vi "lab1AirheaterParams.vi"() -> ()   [LabVIEW 2019]
uses:
  Control 1.ctl
  <vilib>/Simulation/Scripting/Companion Diagram/SimConfigNode/SimParams.ctl
  <vilib>/Simulation/Scripting/Companion Diagram/SimConfigNode/_simSolvers.ctl
  <vilib>/Simulation/Implementation/Shared/SIMSCR Execution Mode.ctl
  <vilib>/Simulation/Param Hierarchy/Typedefs/SIMPH Param Control Actions.ctl
  <vilib>/Simulation/Implementation/Shared/NILVSim_ParamChanged.vi
  <vilib>/Simulation/Implementation/Shared/NILVSIM_BeginStep.vi
  <vilib>/Simulation/Implementation/Shared/NILVSim_Manager.vi
  <vilib>/Utility/error.llb/Clear Errors.vi
  <vilib>/Simulation/Implementation/Shared/NILVSim_FinalizeModel.vi
  <vilib>/DAQmx/write.llb/DAQmx Write (Analog DBL 1Chan 1Samp).vi
  <vilib>/DAQmx/read.llb/DAQmx Read (Analog DBL 1Chan 1Samp).vi
  <vilib>/Simulation/Implementation/Shared/SIM Unbundle Sim Info.vi
  <vilib>/Simulation/Implementation/Shared/NILVSim_Initialize.vi
  <vilib>/Simulation/Utility/Implementation/NILVSim Get Time and IsAcceptedStep.vi
  <vilib>/Simulation/Implementation/Shared/SIMSH Read Queue.vi
  <vilib>/Simulation/Implementation/Shared/NILVSim_GetModelError.vi
  <vilib>/Simulation/Implementation/Shared/SIM Bundle Sim Info.vi
  <vilib>/DAQmx/miscellaneous.llb/DAQmx Fill In Error Info.vi
  <vilib>/Simulation/Implementation/XNodeFramework/SimXNode/SimX.xnode
  subAirheater.vi
  <vilib>/Simulation/Scripting/Companion Diagram/SimConfigNode/SimDog.xnode
  <vilib>/Simulation/Implementation/Shared/NI_SIM_Implementation.lvlib
panel:
  out "Yv [V]":dbl
  in  "stop":bool
  in  "Control Signal [V]":dbl(slide) scale=0.0..5.0
  in  "Time Step [S]":dbl
  out "Temperature Chart":cluster{"data":dbl, "T_out[C]":dbl}(graph)
  out "Control Signal Chart":dbl(graph)
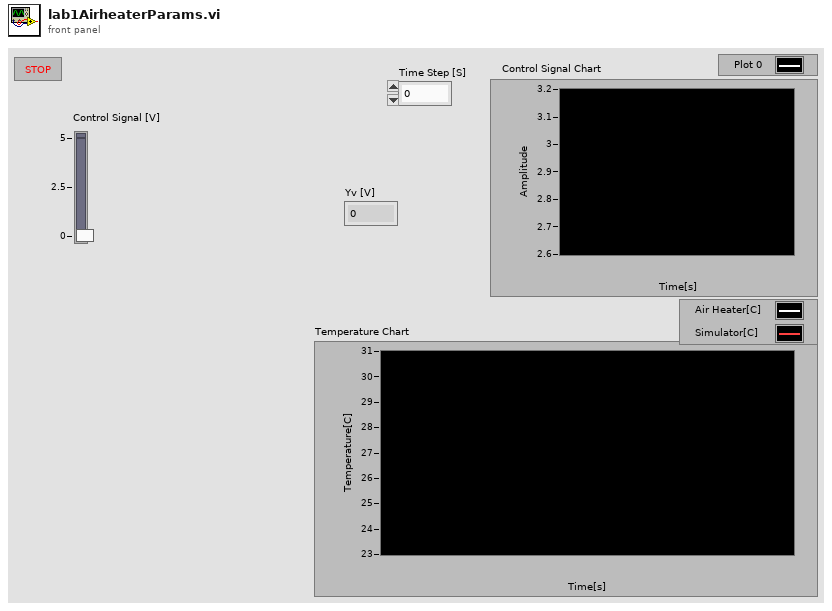
[diagram p1: front panel]
types:
  T1 = typedef "Control 1.ctl" = dbl[]
  T2 = enum16{"Simulate to Completion", "Single Time-Step Simulation (Fixed Step Only)"}
  T3 = typedef "SIMSCR Execution Mode.ctl" = enum16{"Simulate to Completion", "Single Time-Step Simulation (Fixed Step Only)"}
  T4 = typedef "SIMPH Param Control Actions.ctl" = enum16{"get params", "set params"}
  T5 = cluster{"SIMSH Sim Time":dbl, "Operand2":dbl, "Multiplication 3":cluster{"Result":dbl}, "Integrator":cluster{"output":dbl}, "Multiplication 2":cluster{"Result":dbl}, "Summation 2":cluster{"Result":dbl}, "Transport Delay":cluster{"output":dbl}, "Summation":cluster{"Result":dbl}, "Multiplication":cluster{"Result":dbl}}
  T6 = typedef "SimParams.ctl" = cluster{"Initial Time (s)":dbl, "Final Time (s)":dbl, "Step Size (s)":dbl, "ODE Solver":T7, "Minimum Step Size (s)":dbl, "Maximum Step Size (s)":dbl, "Relative Tolerance":dbl, "Absolute Tolerance":dbl, "Software Timing":bool, "Initial Step Size (s)":dbl, "Automatic Fixed Step Size?":bool, "Automatic Discrete Step Size?":bool, "Discrete Step Size (s)":dbl, "Calculate using Time Step":bool, "Solver Wired?":bool, "Prev.Frm.Expected End":u64, "Prev.Frm.Actual End":u64, "Prev.Frm.Finished Late?":bool, "Prev.Iter.Expected End":u64, "Prev.Iter.Actual End":u64, "Prev.Iter.Finished Late?":bool, "Expected Iteration Start":u64, "Actual Iteration Start":u64, "Expected Frame Start":u64, "Actual Frame Start":u64, "Source Name":string, "Name":string, "Period":i64, "Deadline":i64, "Offset":i64, "Start":i64, "Priority":i32, "Timeout":i32, "Processor":i32, "Mode":enum32{"No Change", "Process missed periods, maintain original phase", "Discard missed periods, maintain original phase", "Process missed periods, ignore original phase", "Discard missed periods, ignore original phase"}, "Wakeup reason":enum32{"Normal", "Aborted", "Asynchronous wakeup", "Timing source error", "Timed loop error", "Timeout"}, "Error":errorcluster, "Source Type":string, "Secondary Source Type":string, "Global End Time":u64, "Global Start Time":u64, "Full Solver Reset":bool, "Execution Mode":T3, "Nan/Inf Check":bool, "Custom Solver Library":string, "Solver Is Variable":bool, "custom solver name":string, "Signal Collection Decimation":u32}
  T7 = typedef "_simSolvers.ctl" = enum16{"Runge-Kutta 1 (Euler)", "Runge-Kutta 2", "Runge-Kutta 3", "Runge-Kutta 4", "Runge-Kutta 23 (variable)", "Runge-Kutta 45 (variable)", "BDF (variable)", "Adams-Moulton (variable)", "Rosenbrock (variable)", "Discrete States Only", "SDIRK 4 (variable)", "Radau 5 (variable)", "Radau 9 (variable)", "Radau 13 (variable)", "Radau [Variable Order] (variable)", "Gear's Method (variable)", "Linearizer", "State Query", "Trim Eval", "Custom Solver"}
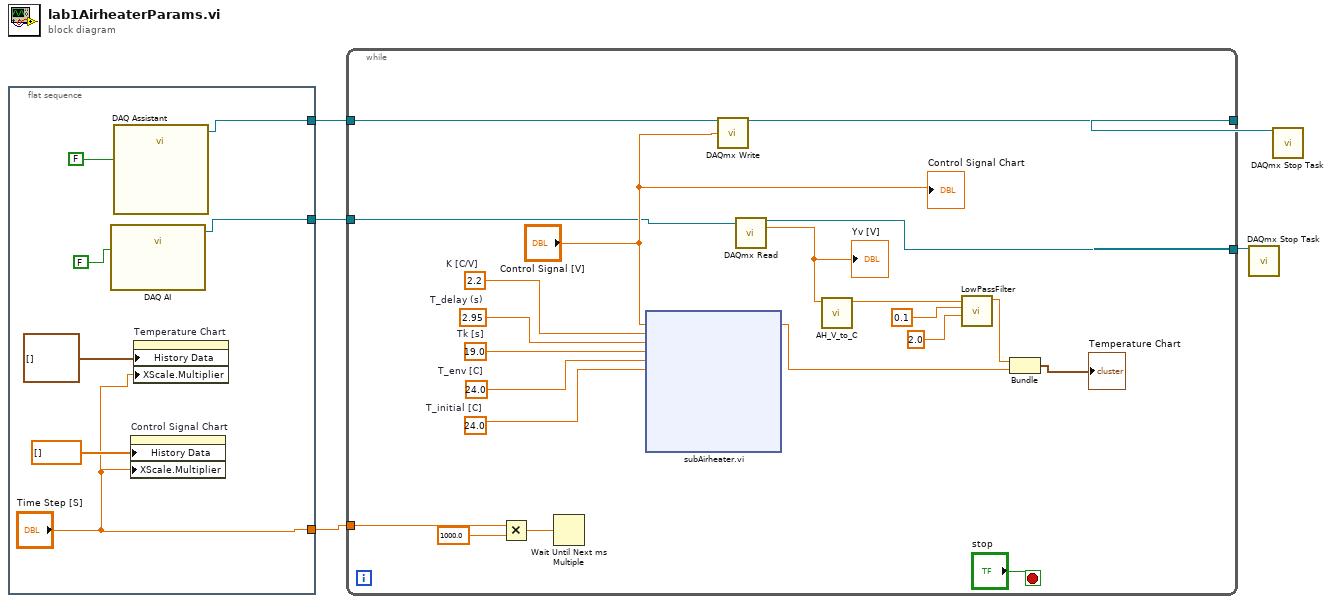
[diagram p0: block diagram]
diagram:
  n1 = flat-sequence {
    tunnel: ["Time Step [S]"] -> w5
    tunnel: [w9] -> w2
    tunnel: [w6] -> w1
    frame #0 {
      n2 = call "DAQ AI"("stop (T)"=FALSE) -> ("task out"=w9:refnum<k21>)  [unwired: 16 in, 2 out]
      n3 = call "DAQ Assistant"("stop (T)"=FALSE) -> ("task out"=w6:refnum<k21>)  [unwired: 17 in, 1 out]
      n4 = property on="Control Signal Chart" class="WFChart (strict)"("History Data"=T1 [], "XScale.Multiplier"="Time Step [S]") -> ()  [unwired: 2 in, 2 out]
      n5 = property on="Temperature Chart" class="WFChart (strict)"("History Data"=cluster{"data":dbl, "T_out[C]":dbl}[] [], "XScale.Multiplier"="Time Step [S]") -> ()  [unwired: 2 in, 2 out]
    }
  }
  n6 = while {
    tunnel: w5 -> [w32]
    tunnel: [w23] -> w4
    tunnel: [w22] -> w3
    tunnel: w2 -> [w14]
    tunnel: w1 -> [w13]
    stop <- "stop" stop-if-true
    w26 = 24.0  # T_initial [C]
    w28 = 2.95  # T_delay (s)
    w29 = 24.0  # T_env [C]
    w27 = 19.0  # Tk [s]
    w30 = 2.2  # K [C/V]
    n7 = Multiply(x=w32, y=1000.0) -> (x*y=w31:dbl)
    n8 = Wait Until Next ms Multiple(millisecond multiple=w31) -> ()  [unwired: 1 out]
    n9 = xnode "subAirheater.vi"("u[V]"="Control Signal [V]", "K[C/V]"=w30, "T_delay (s)"=w28, "Tk [s]"=w27, "T_env [C]"=w29, "T_initial [C]"=w26) -> ("T_out[C]"=w24:dbl)  [unwired: 2 in, 14 out]
    n10 = call-poly <vilib>:"DAQmx Write.vi"("task/channels in"=w13, "data"="Control Signal [V]") -> ("task out"=w23:refnum<k21>)  [unwired: 11 in, 2 out]
    n11 = call-poly <vilib>:"DAQmx Read.vi"("task/channels in"=w14) -> ("task out"=w22:refnum<k21>, "data"=w15:dbl)  [unwired: 12 in, 1 out]
    "Yv [V]" <- w15
    n12 = call "AH_V_to_C.vi"("Vin[1-5V]"=w15) -> ("Tout[C]"=w20:dbl)  [unwired: 10 in]
    n13 = call "LowPassFilter.vi"("Tf[s]"=2.0, "Ts[s]"=0.1, "u_k"=w20) -> ("output variable"=w17:dbl)  [unwired: 8 in]
    n14 = Bundle("output variable"=w17, "T_out[C]"=w24) -> (→"Temperature Chart":cluster{"output variable":dbl, "T_out[C]":dbl})  [unwired: 1 in]
    "Control Signal Chart" <- "Control Signal [V]"
  }
  n15 = call <vilib>:"DAQmx Stop Task.vi"("task/channels in"=w3) -> ()  [unwired: 13 in, 2 out]
  n16 = call <vilib>:"DAQmx Stop Task.vi"("task/channels in"=w4) -> ()  [unwired: 13 in, 2 out]
